vi "remove_terminator_from_begin.vi"(11 "BSONbytes":u8[](array[numeric])) -> (3 "restOfBytes":u8[](array[numeric]))   [LabVIEW 2015, in "BSON_convertors_Library.lvlib"]
uses:
  BSON_convertors_Library.lvlib
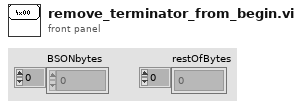
[diagram p1: front panel]
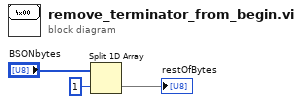
[diagram p0: block diagram]
diagram:
  n1 = Split 1D Array(array="BSONbytes", index=1) -> (second subarray=→"restOfBytes":u8[])  [unwired: 1 out]
